vi "3 Totes Strafe.vi"   [LabVIEW 2014]
types:
  T1 = enum16{"Move Forward", "Move Backward", "Strafe Right", "Strafe Left"}
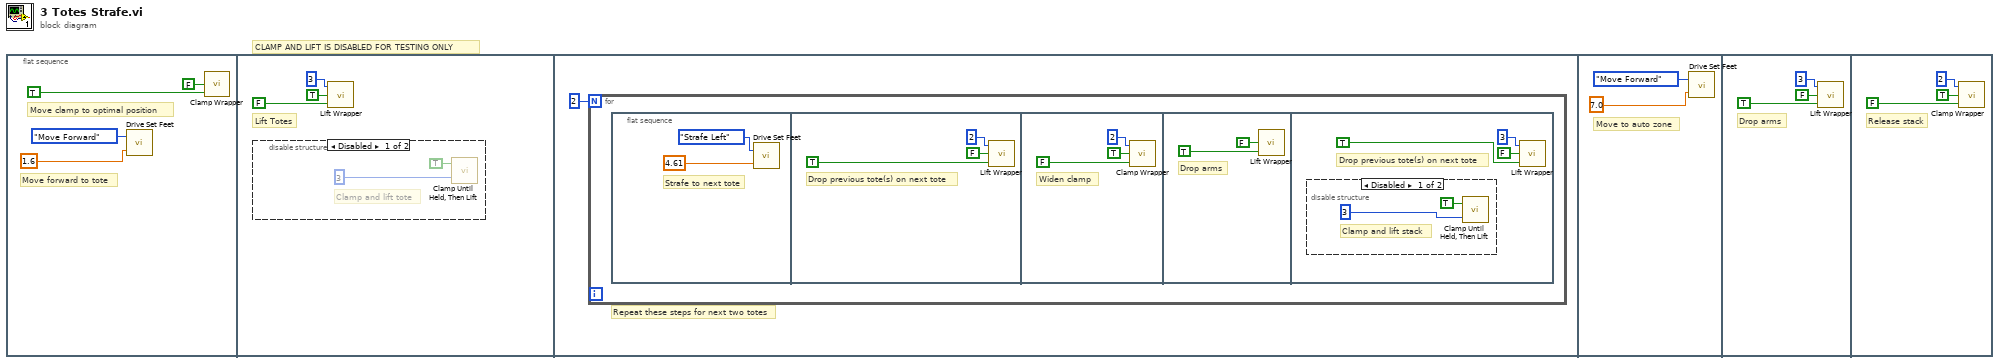
[diagram p0: block diagram]
diagram:
  # "CLAMP AND LIFT IS DISABLED FOR TESTING ONLY"
  n1 = flat-sequence {
    frame #0 {
      # "Move clamp to optimal position"
      # "Move forward to tote"
      n2 = call "Drive Set Feet.vi"("Feet"=1.6, "Direction"=T1."Move Forward") -> ()  [unwired: 1 out]
      n3 = call "Clamp Wrapper.vi"("In"=TRUE, "Out"=FALSE) -> ()  [unwired: 1 in]
    }
    frame #1 {
      # "Lift Totes"
      n4 = disable-structure shown="Disabled" {
        frame Disabled {
          # "Clamp and lift tote"
          n5 = call "Clamp Until Held, Then Lift.vi"("Iterations"=3, "Clamp + Lift"=TRUE) -> ()  [unwired: 1 in]
        }
        frame Enabled {
        }
      }
      n6 = call "Lift Wrapper.vi"("Down"=FALSE, "Up"=TRUE, "Iterations"=3) -> ()
    }
    frame #2 {
      # "Repeat these steps for next two totes"
      n7 = for {
        N: 2 -> [_]
        n8 = flat-sequence {
          frame #0 {
            # "Strafe to next tote"
            n9 = call "Drive Set Feet.vi"("Feet"=4.61, "Direction"=T1."Strafe Left") -> ()  [unwired: 1 out]
          }
          frame #1 {
            # "Drop previous tote(s) on next tote"
            n10 = call "Lift Wrapper.vi"("Down"=TRUE, "Up"=FALSE, "Iterations"=2) -> ()
          }
          frame #2 {
            # "Widen clamp"
            n11 = call "Clamp Wrapper.vi"("In"=FALSE ("In or Out"), "Out"=TRUE, "Iterations"=2) -> ()
          }
          frame #3 {
            # "Drop arms"
            n12 = call "Lift Wrapper.vi"("Down"=TRUE ("Up or Down"), "Up"=FALSE) -> ()  [unwired: 1 in]
          }
          frame #4 {
            # "Drop previous tote(s) on next tote"
            n13 = disable-structure shown="Disabled" {
              frame Disabled {
                # "Clamp and lift stack"
                n14 = call "Clamp Until Held, Then Lift.vi"("Iterations"=3, "Clamp + Lift"=TRUE) -> ()  [unwired: 1 in]
              }
              frame Enabled {
              }
            }
            n15 = call "Lift Wrapper.vi"("Down"=TRUE, "Up"=FALSE, "Iterations"=3) -> ()
          }
        }
      }
    }
    frame #3 {
      # "Move to auto zone"
      n16 = call "Drive Set Feet.vi"("Feet"=7.0, "Direction"=T1."Move Forward") -> ()  [unwired: 1 out]
    }
    frame #4 {
      # "Drop arms"
      n17 = call "Lift Wrapper.vi"("Down"=TRUE ("Up or Down"), "Up"=FALSE, "Iterations"=3) -> ()
    }
    frame #5 {
      # "Release stack"
      n18 = call "Clamp Wrapper.vi"("In"=FALSE ("In or Out"), "Out"=TRUE, "Iterations"=2) -> ()
    }
  }
